vi "SetAttributeViInt32_SA-Limit_Mask.vi"(7 "AttributeValue":i32 format="%.0g", 8 "error in (no error)":errorcluster {"code" format="%.0x"}, 9 "AttributeID":u32(ring)=1150614 items=["SA_LIMIT_AMPLITUDE_INTERPOLATOR"=1150614, "SA_LIMIT_DOMAIN"=1150620, "SA_LIMIT_FREQUENCY_INTERPOLATOR"=1150623, "SA_LIMIT_MODE"=1150626, "SA_LIMIT_TEST_TRACE"=1150629, "SA_LIMIT_TYPE"=1150630, "SA_SEMASK_AVERAGE_COUNT"=1150359, "SA_SEMASK_DISPLAY_VIEW"=1150395, "SA_SEMASK_DISPLAY_VIEW_SELECTION"=1150396, "SA_SEMASK_DISPLAY_WINDOWX_REF_POSITION"=1150816, "SA_SEMASK_DISPLAY_WINDOWY_REF_POSITION"=1150386, "SA_SEMASK_MARKER_ACTIVE_MARKER"=1150399, "SA_SEMASK_MARKER_TYPE"=1150408, "SA_SEMASK_MEASUREMENT_TYPE"=1150358, "SA_SEMASK_OFFSET_DETECTOR_TYPE"=1150407, "SA_SEMASK_OFFSET_TYPE"=1150420, "SA_SEMASK_REFERENCECHANNEL_DETECTOR_TYPE"=1150367, "SA_SEMASK_SWEEPCOUPLING_BANDWIDTH_SHAPE"=1150370, "SA_SEMASK_SWEEPCOUPLING_MEASUREMENT_TYPE"=1150818, "SA_SEMASK_SWEEPCOUPLING_SWEEP_TYPE_AUTO_RULES"=1150820, "SA_SEMASK_TRACES_TYPE"=1150780, "SA_SEMASK_TRIGGER_SOURCE"=1150357], 10 "RepCapIdentifier":string, 11 "instrument handle":refnum<k15>) -> (0 "error out":errorcluster {"code" format="%.0x"}, 3 "instrument handle out":refnum<k15>)   [LabVIEW 2009, in "Keysight XSAn.lvlib"]
doc: "Sets an Int32 attribute from the instrument driver.\nThe following Attributes are supported:\n\nSA_LIMIT_AMPLITUDE_INTERPOLATOR\nSA_LIMIT_DOMAIN\nSA_LIMIT_FREQUENCY_INTERPOLATOR\nSA_LIMIT_MODE\nSA_LIMIT_TEST_TRACE\nSA_LIMIT_TYPE\nSA_SEMASK_AVERAGE_COUNT\nSA_SEMASK_DISPLAY_VIEW\nSA_SEMASK_DISPLAY_VIEW_SELECTION\nSA_SEMASK_DISPLAY_WINDOWX_REF_POSITION \nSA_SEMASK_DISPLAY_WINDOWY_REF_POSITION\nSA_SEMASK_MARKER_ACTIVE_MARKER\nSA_SEMASK_MARKER_TYPE\nSA_SEMASK_MEASUREMENT_TYPE\nSA_SEMASK_OFFSET_DETECTOR_TYPE\nSA_SEMASK_OFFSET_TYPE\nSA_SEMASK_REFERENCECHANNEL_DETECTOR_TYPE\nSA_SEMASK_SWEEPCOUPLING_BANDWIDTH_SHAPE\nSA_SEMASK_SWEEPCOUPLING_MEASUREMENT_TYPE\nSA_SEMASK_SWEEPCOUPLING_SWEEP_TYPE_AUTO_RULES \nSA_SEMASK_TRACES_TYPE\nSA_SEMASK_TRIGGER_SOURCE"
uses:
  <instrlib>/Keysight XSAn/Keysight XSAn.lvlib
  AgXSAn.dll
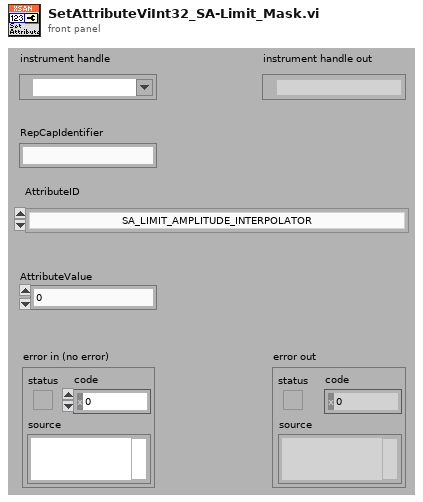
[diagram p1: front panel]
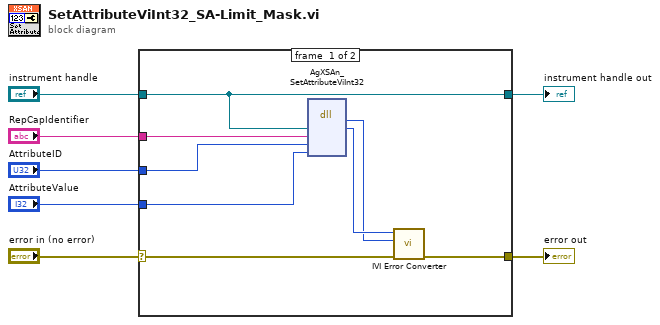
[diagram p0: block diagram]
diagram:
  n1 = case shown="No Error" "error in (no error)" {
    selector: "error in (no error)" -> [w13 w17]
    tunnel: [w12 w17] -> w7
    tunnel: "instrument handle" -> [w8 w16]
    tunnel: "RepCapIdentifier" -> [w11 _]
    tunnel: "AttributeID" -> [w10 _]
    tunnel: "AttributeValue" -> [w9 _]
    tunnel: [w8 w16] -> w1
    frame #0 {
      n2 = dll-call lib="AgXSAn**.dll" fn="AgXSAn_SetAttributeViInt32"("Vi"=w8, "RepCapIdentifier"=w11, "AttributeID"=w10, "AttributeValue"=w9) -> ("return type"=w14:i32, "Vi"=w15:u32)  [unwired: 6 in, 2 out]
      n3 = call <instrlib>:"IVI Error Converter.vi"("error in (no error)"=w13, "IVI error code (0)"=w14, "instrument handle"=w15) -> ("error out"=w12:errorcluster)  [unwired: 7 in, 1 out]
    }
    frame #1 {
    }
  }
  "error out" <- w7
  "instrument handle out" <- w1
